vi "통신sub.vi"(0 "FGV 상태":enum16{"쓰기", "읽기", ""}(ring), 1 "입력":dbl) -> (7 "출력":dbl)   [LabVIEW 2020]
panel:
  in  "정지":bool
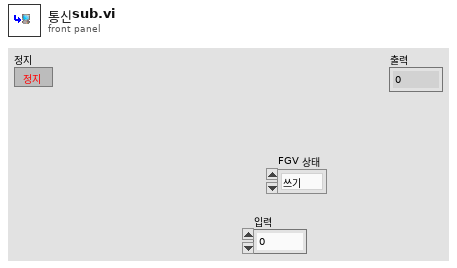
[diagram p1: front panel]
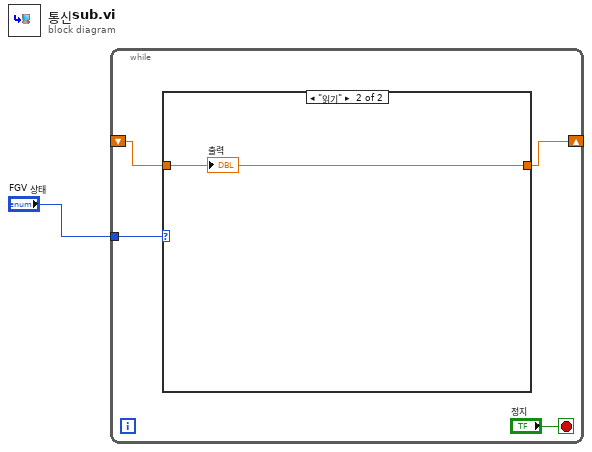
[diagram p0: block diagram]
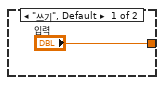
[diagram p2: hidden frame]
diagram:
  n1 = while {
    tunnel: "FGV 상태" -> [w5]
    shift-right: [w4] -> _
    shift-left: _ -> [w3]
    stop <- "정지" stop-if-true
    n2 = case shown="\"읽기\"" w5 {
      tunnel: ["입력" w7] -> w4
      tunnel: w3 -> [_ w7]
      frame "쓰기", Default {
      }
      frame "읽기" {
        "출력" <- w7
      }
    }
  }
